vi "Get Time.vi"(8 "error in (no error)":errorcluster, 11 "Board Game in":refnum<class "Board Game.lvclass">) -> (0 "error out":errorcluster, 3 "Time":u32)   [LabVIEW 2021, in "Board Game.lvclass"]
uses:
  Board Game.lvclass
  Board Game.lvclass/Board Game.ctl
  Snake_class/Snake.lvclass/Snake.ctl
  Snake_class/Read Star.vi
  Snake_class/Snake.lvclass
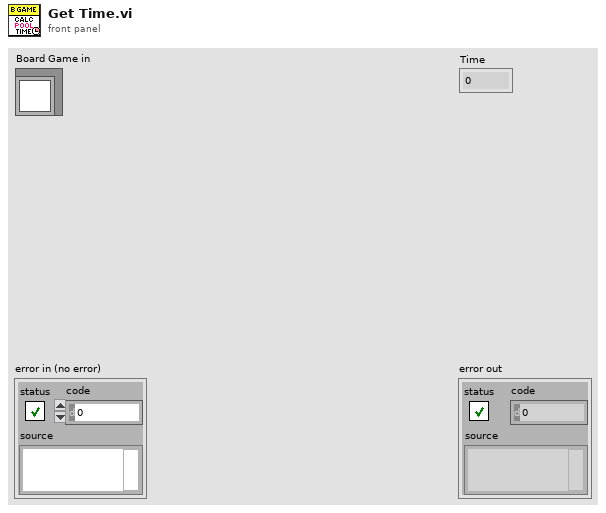
[diagram p1: front panel]
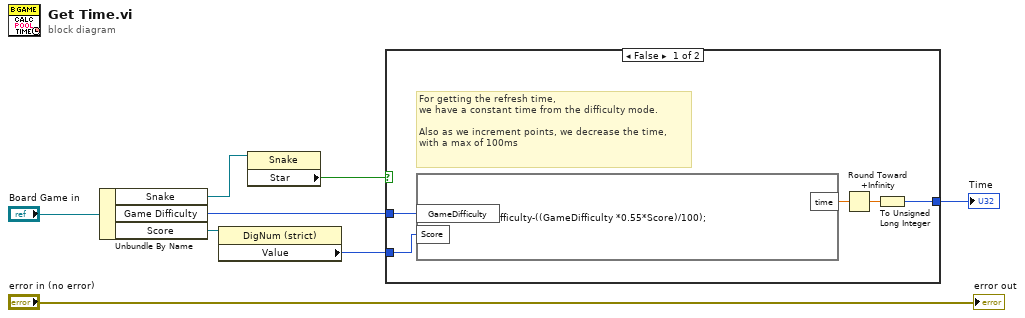
[diagram p0: block diagram]
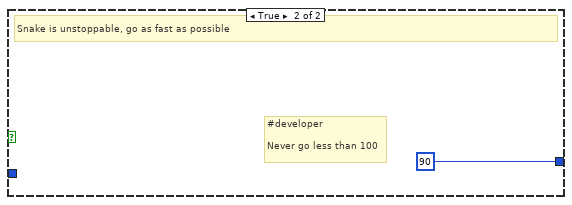
[diagram p2: hidden frame]
diagram:
  n1 = Unbundle By Name("Board Game in") -> ("Snake"=w2:refnum<class "Snake.lvclass">, "Game Difficulty"=w6:u32, "Score"=w4:refnum<vi>)
  n2 = property class="DigNum (strict)"(reference=w4) -> ("Value"=w3:u16)  [unwired: 1 in, 2 out]
  n3 = property class="Snake"(reference=w2) -> ("Star"=w1:bool)  [unwired: 1 in, 2 out]
  n4 = case shown="False" w1 {
    tunnel: w6 -> [w13 _]
    tunnel: [w10 u32 90] -> w5
    tunnel: w3 -> [w9 _]
    frame False {
      # "For getting the refresh time, \nwe have a constant time from the difficulty mode. \n\nAlso as we increment points, we decrease the time, \nwith a max of 100ms"
      n5 = formula code="time = GameDifficulty-((GameDifficulty *0.55*Score)/100);"("GameDifficulty"=w13, "Score"=w9) -> ("time"=w12:dbl)
      n6 = Round Toward +Infinity(x=w12) -> (ceil(x): smallest int >= x=w11:dbl)
      n7 = To Unsigned Long Integer(number=w11) -> (unsigned 32bit integer=w10:u32)
    }
    frame True {
      # "#developer\n\nNever go less than 100"
      # "Snake is unstoppable, go as fast as possible"
    }
  }
  "Time" <- w5
  "error out" <- "error in (no error)"
